vi "Lookup Target Channels.vi"(6 "VolatusAPI":refnum<class "VolatusAPI.lvclass">, 8 "error in (no error)":errorcluster, 11 "LoggingControl in":refnum<class "GroupLoggingControl.lvclass">) -> (0 "error out":errorcluster, 3 "LoggingControl out":refnum<class "GroupLoggingControl.lvclass">)   [LabVIEW 2020, in "VolatusGUIElements.lvlib" / "GroupLoggingControl.lvclass"]
uses:
  GroupLoggingControl.lvclass
  Volatus/VolatusAPI/VolatusAPI.lvclass
  VolatusConfig/Meta Name.ctl
  Volatus/VolatusAPI/VolatusAPI.lvclass/VolatusAPI.ctl
  GroupLoggingControl.lvclass/GroupLoggingControl.ctl
  VolatusConfig/VolatusConfigElement/VolatusConfigElement.lvclass/VolatusConfigElement.ctl
  lv-vecto/Vecto/Channel STR/Channel STR.lvclass/Channel STR.ctl
  VolatusConfig/VolatusConfigElement/Element.vi
  lv-vecto/Vecto/Channel STR/Init.vi
  VolatusConfig/Node/Node Config.lvclass
  C:/dev/lv20CE/relink/lv-volatus/VolatusConfig/VolatusConfigElement/VolatusConfigElement.lvclass
  lv-cdm/CDM-Config/Config Element/Owner.vi
  lv-cdm/CDM-Config/Config Manager/Lookup Descendant.vi
  lv-cdm/CDM-Config/Config Filter/Config Lookup.lvclass
  lv-vecto/Vecto/Channel STR/Channel STR.lvclass
  VolatusConfig/Cluster/Cluster Config.lvclass
  VolatusConfig/VolatusConfigElement/VolatusConfigElement.lvclass
  VolatusConfig/Channel/Channel Config.lvclass
  lv-vecto/Vecto/Group STR/Group STR.lvclass
  lv-vecto/Vecto/Group/Group.lvclass
  VolatusConfig/VolatusConfig.lvlib
  lv-cdm/CDM-Config/Config Element/Config Element.lvclass
  lv-vecto/Vecto/Group DBL/Group DBL.lvclass
  C:/dev/lv20CE/relink/lv-vecto/Vecto/Group/Group.lvclass
  C:/dev/lv20CE/relink/lv-vecto/Vecto/Group DBL/Group DBL.lvclass
  C:/dev/lv20CE/relink/lv-vecto/Vecto/Group STR/Group STR.lvclass
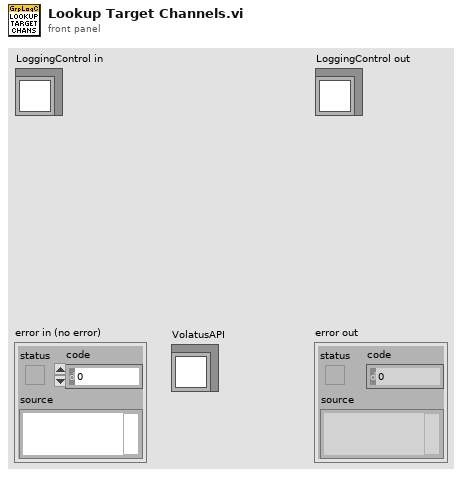
[diagram p1: front panel]
types:
  T1 = typedef "VolatusConfig.lvlib/Meta Name.ctl" = enum16{"VL_Type", "VL_Node_IP", "VL_Node_Type", "VL_Task_Type", "VL_Group_Type", "VL_Channel_Type", "VL_Channel_DataType", "VL_Config_Version", "VL_Overlay_Type", "VL_Config_Hash"}
  T2 = typedef "VolatusGUIElements.lvlib/GroupLoggingControl.lvclass/Target Info.ctl" = cluster{"Node":string, "Node Color":u32, "Groups":T3[]}
  T3 = typedef "VolatusGUIElements.lvlib/GroupLoggingControl.lvclass/Log Group.ctl" = cluster{"Status":T4, "Command Info":T5, "Logging":bool, "State":string}
  T4 = typedef "VolatusGUIElements.lvlib/GroupLoggingControl.lvclass/Log Group Status.ctl" = cluster{"Group":string, "Group Color":u32, "Button":bool}
  T5 = typedef "VolatusGUIElements.lvlib/GroupLoggingControl.lvclass/Command Info.ctl" = cluster{"Commanding":bool, "Cmd Time":dbl, "Group ID":string}
  T6 = map{string, refnum<class "Config Element.lvclass">}
  T7 = typedef "VectoConfig.lvlib/Channel Info.ctl" = cluster{"Name":string, "Group":string, "Owning Node":string, "Owning Task":string, "Resource":string}
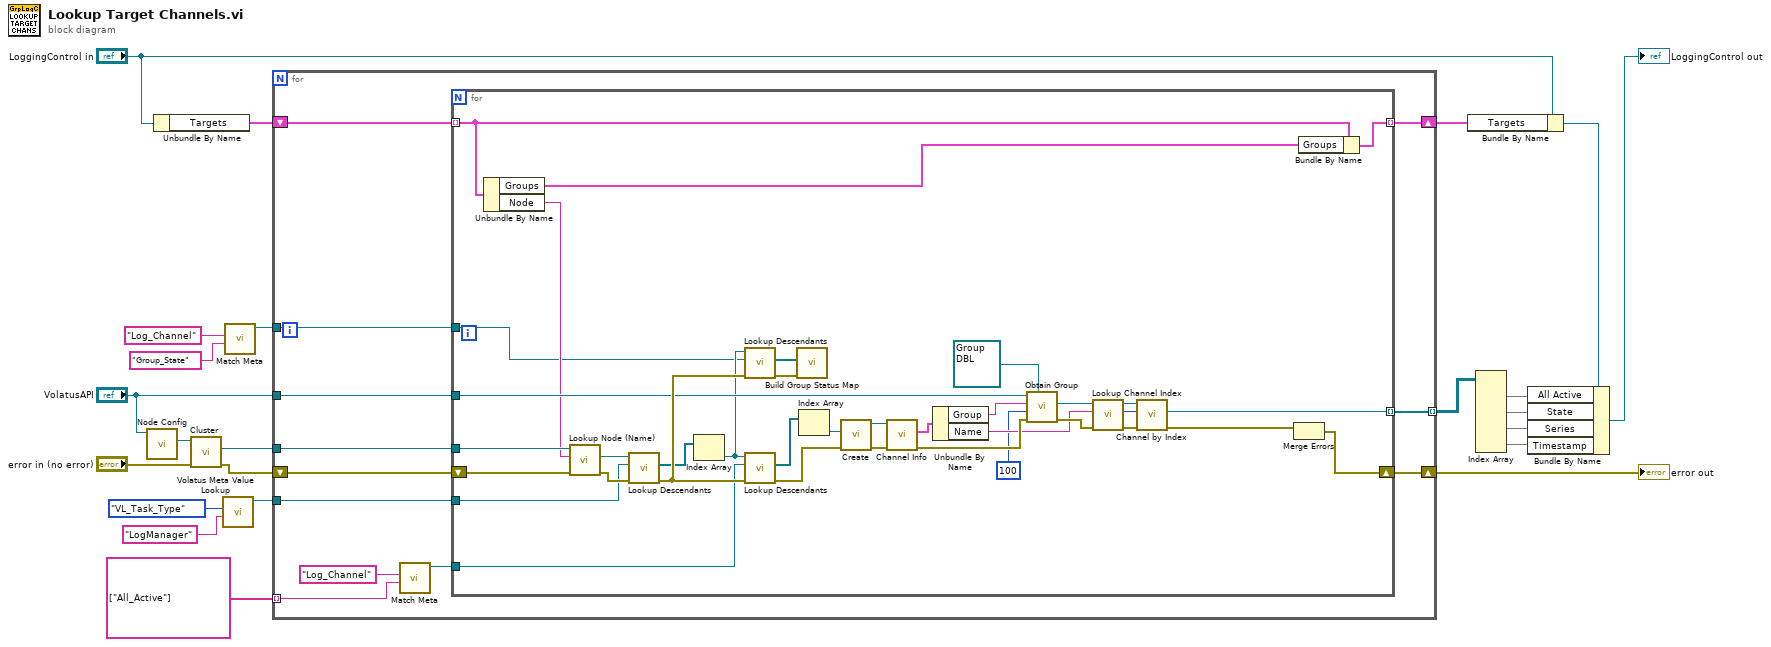
[diagram p0: block diagram]
diagram:
  n1 = call "Node Config.vi"("VolatusAPI in"="VolatusAPI") -> ("Node Config"=w22:refnum<class "Node Config.lvclass">)  [unwired: 9 in, 1 out]
  n2 = Unbundle By Name("LoggingControl in") -> ("Targets"=w20:T2[])
  n3 = call "Cluster.vi"("error in (no error)"="error in (no error)", "Node in"=w22) -> ("error out"=w19:errorcluster, "Cluster"=w21:refnum<class "Cluster Config.lvclass">)  [unwired: 7 in, 1 out]
  n4 = call "Volatus Meta Value Lookup.vi"("Value"="LogManager", "Meta Name"=Meta_Name."VL_Task_Type") -> ("Config Lookup out"=w4:refnum<class "Config Lookup.lvclass">)  [unwired: 8 in, 1 out]
  n5 = call "Match Meta.vi"("Value (Any)"="Group_State" ("Name"), "Name"="Log_Channel") -> ("Config Lookup out"=w1:refnum<class "Config Lookup.lvclass">)  [unwired: 8 in, 1 out]
  n6 = for {
    tunnel: w21 -> [w35]
    tunnel: "VolatusAPI" -> [w32]
    tunnel: [w31] -> w14 mode=indexing
    shift-right: [w30] -> w9
    shift-left: w19 -> [w33]
    tunnel: string[] ["All_Active"] -> [w27] mode=indexing
    shift-right: [w26] -> w7
    shift-left: w20 -> [w34]
    tunnel: w4 -> [w25]
    tunnel: w1 -> [w24]
    n7 = call "Match Meta.vi"("Value (Any)"=w27, "Name"="Log_Channel") -> ("Config Lookup out"=w28:refnum<class "Config Lookup.lvclass">)  [unwired: 8 in, 1 out]
    n8 = for {
      tunnel: w35 -> [w71]
      tunnel: w34 -> [w55] mode=indexing
      tunnel: w28 -> [w49]
      shift-right: [w39] -> w30
      shift-left: w33 -> [w70]
      tunnel: w32 -> [w66]
      tunnel: [w62] -> w31 mode=indexing
      tunnel: [w54] -> w26 mode=indexing
      tunnel: w25 -> [w51]
      tunnel: w24 -> [w44]
      n9 = Unbundle By Name(w55) -> ("Groups"=w36:T3[], "Node"=w56:string)
      n10 = call "Lookup Node (Name).vi"("error in (no error)"=w70, "Node Name"=w56, "Cluster in"=w71) -> ("error out"=w52:errorcluster, "Node"=w53:refnum<class "Node Config.lvclass">)  [unwired: 6 in, 1 out]
      n11 = call "Lookup Descendants.vi"("error in (no error)"=w52, "Lookup"=w51, "VolatusConfigElement in"=w53) -> ("error out"=w74:errorcluster, "Descendants"=w50:refnum<class "Config Element.lvclass">[])  [unwired: 6 in, 1 out]
      n12 = Index Array(array=w50) -> (element=w46:refnum<class "Config Element.lvclass">)  [unwired: 1 in]
      n13 = call "Lookup Descendants.vi"("error in (no error)"=w74, "Lookup"=w44, "Config Element in"=w46) -> ("error out"=w43:errorcluster, "Descendants"=w42:refnum<class "Config Element.lvclass">[])  [unwired: 6 in, 1 out]
      n14 = call "Lookup Descendants.vi"("error in (no error)"=w74, "Lookup"=w49, "Config Element in"=w46) -> ("error out"=w47:errorcluster, "Descendants"=w48:refnum<class "Config Element.lvclass">[])  [unwired: 6 in, 1 out]
      n15 = call "Build Group Status Map.vi"("error in (no error)"=w43, "Descendants"=w42) -> ("error out"=w41:errorcluster, "Map"=w40:T6)  [unwired: 8 in]
      n16 = Index Array(array=w48) -> (element=w69:refnum<class "Config Element.lvclass">)  [unwired: 1 in]
      n17 = call "Create.vi"("error in (no error)"=w47, "Element"=w69) -> ("error out"=w67:errorcluster, "Channel out"=w68:refnum<class "Channel Config.lvclass">)  [unwired: 8 in]
      n18 = call "Channel Info.vi"("error in (no error)"=w67, "Channel in"=w68) -> ("error out"=w73:errorcluster, "Channel Info"=w65:T7)  [unwired: 7 in, 1 out]
      n19 = Unbundle By Name(w65) -> ("Group"=w63:string, "Name"=w58:string)
      n20 = call "Obtain Group.vi"("Group Type (Abstract)"=refnum<class "Group DBL.lvclass"> refnum ("Vecto.lvlib:StringGroup.lvclass"), "error in (no error)"=w73, "Timeout ms (5000)"=u32 100, "Group Name"=w63, "VolatusAPI in"=w66) -> ("error out"=w72:errorcluster, "Group"=w45:refnum<class "Group DBL.lvclass">)  [unwired: 4 in, 1 out]
      n21 = call "Lookup Channel Index.vi"("error in (no error)"=w72, "Channel Name"=w58, "Group in"=w45) -> ("error out"=w57:errorcluster, "Index"=w59:i32, "Group out"=w60:refnum<class "Group DBL.lvclass">)  [unwired: 6 in]
      n22 = call "Channel by Index.vi"("error in (no error)"=w57, "Index"=w59, "StringGroup in"=w60) -> ("error out"=w61:errorcluster, "StringChannel"=w62:refnum<class "Channel STR.lvclass">)  [unwired: 6 in, 1 out]
      n23 = Merge Errors(w61) -> (w39:errorcluster, w38:errorcluster[])
      n24 = Bundle By Name(cluster=w55, "Groups"=w36) -> (w54:T2)
    }
  }
  "error out" <- w9
  n25 = Bundle By Name(cluster="LoggingControl in", "Targets"=w7) -> (w8:refnum<class "GroupLoggingControl.lvclass">)
  n26 = Index Array(array=w14) -> (element #1=w13:refnum<class "Channel STR.lvclass">[], element #2=w12:refnum<class "Channel STR.lvclass">[], element #3=w11:refnum<class "Channel STR.lvclass">[], element #4=w10:refnum<class "Channel STR.lvclass">[])  [unwired: 8 in]
  n27 = Bundle By Name(cluster=w8, "All Active"=w13, "State"=w12, "Series"=w11, "Timestamp"=w10) -> (→"LoggingControl out":refnum<class "GroupLoggingControl.lvclass">)
